vi "Scripting_SaveUpdateSubVIs.vi"(8 "error in (no error)":errorcluster, 11 "VI Refnum":refnum<vi>) -> (0 "error out":errorcluster)   [LabVIEW 2014]
uses:
  <vilib>/Utility/traverseref.llb/TRef TravTarget.ctl
  <vilib>/Utility/traverseref.llb/VI Scripting - Traverse.lvlib
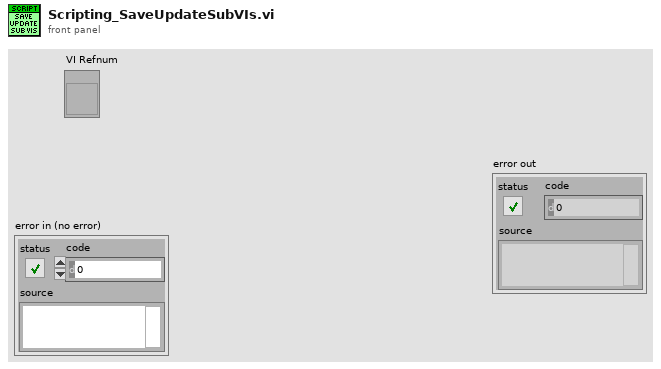
[diagram p1: front panel]
types:
  T1 = typedef "TRef TravTarget.ctl" = enum16{"FP", "BD", "Other"}
  T2 = enum32{"invalid lock state", "Not Locked", "Locked (No Password)", "Password-protected"}
  T3 = enum32{"not a typedef", "typedef", "strict typedef", "class private data"}
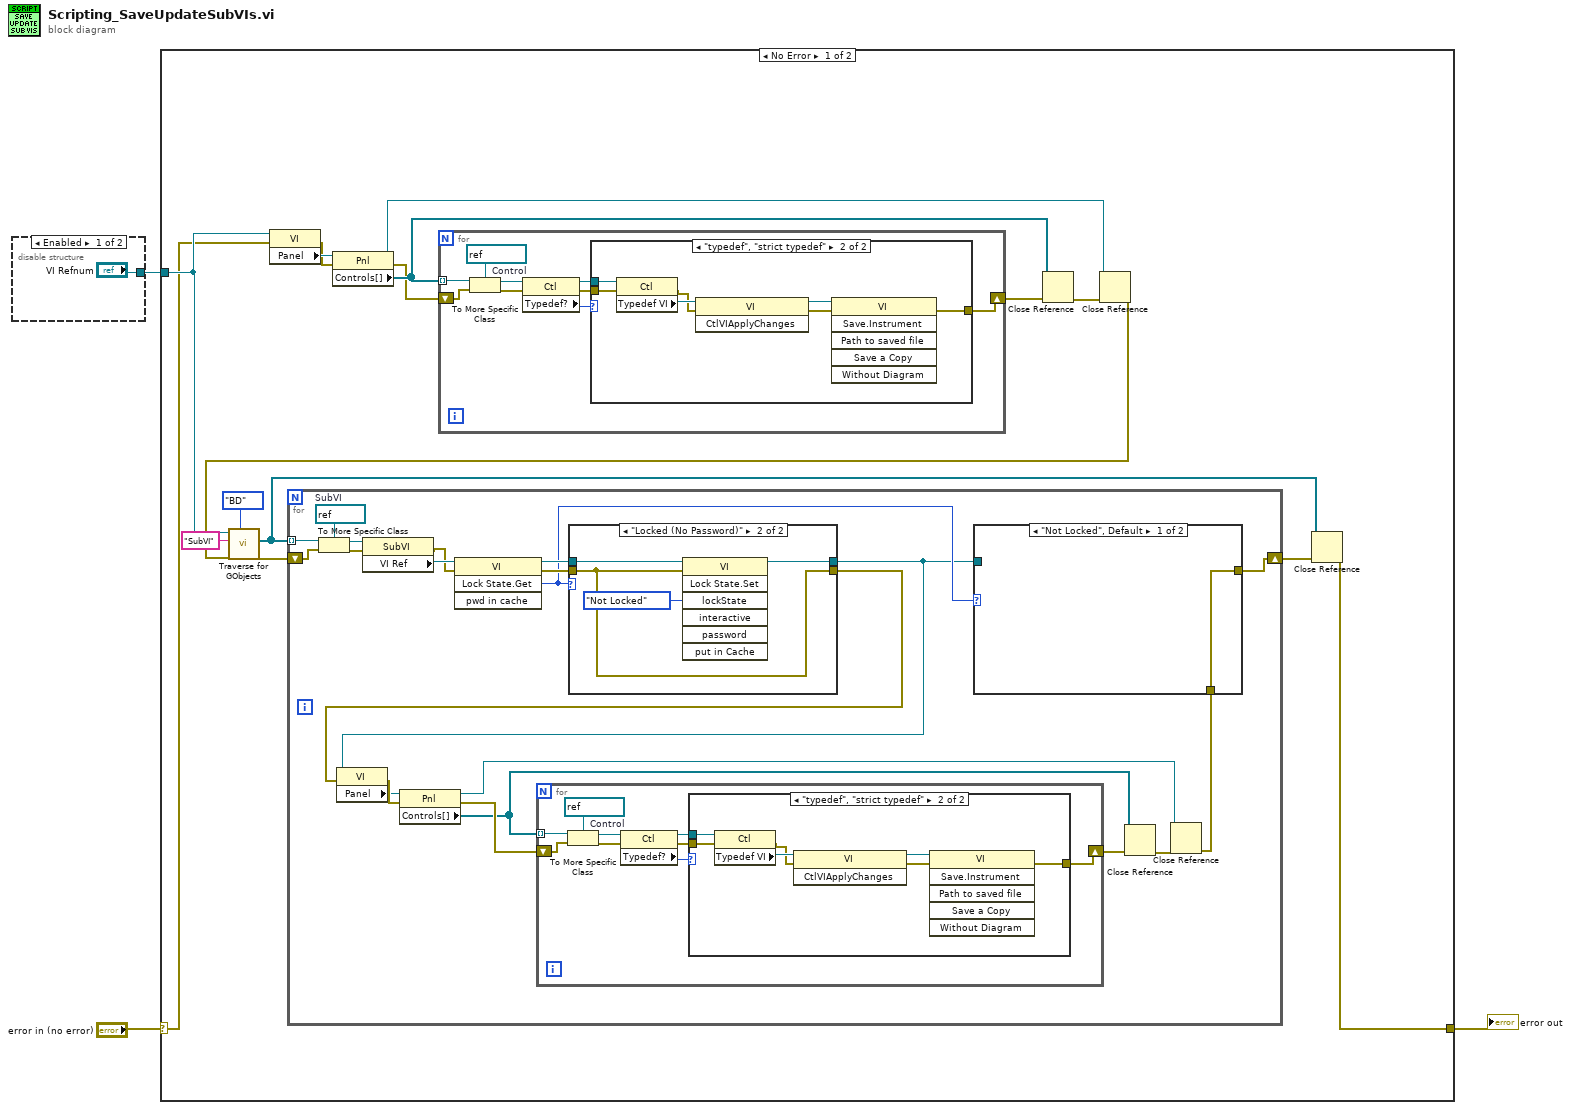
[diagram p0: block diagram]
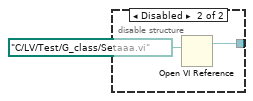
[diagram p2: hidden frame]
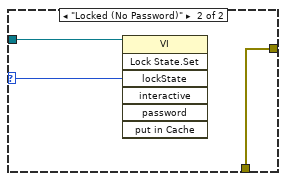
[diagram p3: hidden frame]
diagram:
  n1 = disable-structure shown="Enabled" {
    disable-tunnel: ["VI Refnum" w6] -> w1
    frame Enabled {
    }
    frame Disabled {
      n2 = Open VI Reference(vi path=path "C:/LV/Test/G_class/Setaaa.vi") -> (vi reference=w6:refnum<vi>)  [unwired: 5 in, 1 out]
    }
  }
  n3 = case shown="No Error" "error in (no error)" {
    selector: "error in (no error)" -> [w10 w88]
    tunnel: [w16 w88] -> w2
    tunnel: w1 -> [w15 _]
    frame No Error {
      n4 = property class="VI"(reference=w15, error in=w10) -> (error out=w11:errorcluster, "Panel"=w14:refnum<vi>)  [unwired: 1 out]
      n5 = property class="Pnl"(reference=w14, error in=w11) -> (reference out=w9:refnum<vi>, error out=w12:errorcluster, "Controls[]"=w13:refnum<vi>[])
      n6 = for {
        tunnel: w13 -> [w78] mode=indexing
        shift-right: [w71] -> w22
        shift-left: w12 -> [w75]
        w79 = refnum<vi> refnum  # Control
        n7 = To More Specific Class(target class=w79, reference=w78, error in=w75) -> (specific class reference=w77:refnum<vi>, error out=w76:errorcluster)
        n8 = property class="Ctl"(reference=w77, error in=w76) -> (reference out=w73:refnum<vi>, error out=w72:errorcluster, "Typedef?"=w74:T3)
        n9 = case shown="\"typedef\", \"strict typedef\"" w74 {
          tunnel: w73 -> [_ w87]
          tunnel: w72 -> [w80 w86]
          tunnel: [w80 w81] -> w71
          frame "not a typedef", Default {
          }
          frame "typedef", "strict typedef" {
            n10 = property class="Ctl"(reference=w87, error in=w86) -> (error out=w82:errorcluster, "Typedef VI"=w85:refnum<vi>)  [unwired: 1 out]
            n11 = invoke class="VI" method="CtlVIApplyChanges"(reference=w85, error in=w82) -> (reference out=w84:refnum<vi>, error out=w83:errorcluster)  [unwired: 1 in, 1 out]
            n12 = invoke class="VI" method="Save.Instrument"(reference=w84, error in=w83) -> (error out=w81:errorcluster)  [unwired: 4 in, 5 out]
          }
        }
      }
      n13 = Close Reference(reference=w13, error in (no error)=w22) -> (error out=w8:errorcluster)
      n14 = Close Reference(reference=w9, error in (no error)=w8) -> (error out=w7:errorcluster)
      n15 = call <vilib>:"Traverse for GObjects.vi"("Traverse Target"=TRef_TravTarget."BD", "error in (no error)"=w7, "Class Name"="SubVI", "VI Refnum"=w15) -> ("error out"=w19:errorcluster, "References"=w21:refnum<vi>[])  [unwired: 4 in, 2 out]
      n16 = for {
        tunnel: w21 -> [w42] mode=indexing
        shift-right: [w32] -> w20
        shift-left: w19 -> [w41]
        w43 = refnum<vi> refnum  # SubVI
        n17 = To More Specific Class(target class=w43, reference=w42, error in=w41) -> (specific class reference=w40:refnum<vi>, error out=w39:errorcluster)
        n18 = property class="SubVI"(reference=w40, error in=w39) -> (error out=w36:errorcluster, "VI Ref"=w38:refnum<vi>)  [unwired: 1 out]
        n19 = invoke class="VI" method="Lock State.Get"(reference=w38, error in=w36) -> (reference out=w37:refnum<vi>, error out=w35:errorcluster, "Get Lock State"=w33:T2)  [unwired: 2 in, 1 out]
        n20 = case shown="\"Locked (No Password)\"" w33 {
          tunnel: w37 -> [w65 w70]
          tunnel: w35 -> [w66 w67]
          tunnel: [w65 w68] -> w26
          tunnel: [w66 w67] -> w29
          frame "Not Locked", Default {
          }
          frame "Locked (No Password)" {
            n21 = invoke class="VI" method="Lock State.Set"(reference=w70, error in=w67, "lockState"=T2."Not Locked" ("Lock State")) -> (reference out=w68:refnum<vi>)  [unwired: 4 in, 6 out]
          }
        }
        n22 = property class="VI"(reference=w26, error in=w29) -> (error out=w31:errorcluster, "Panel"=w30:refnum<vi>)  [unwired: 1 out]
        n23 = property class="Pnl"(reference=w30, error in=w31) -> (reference out=w23:refnum<vi>, error out=w28:errorcluster, "Controls[]"=w27:refnum<vi>[])
        n24 = for {
          tunnel: w27 -> [w55] mode=indexing
          shift-right: [w48] -> w34
          shift-left: w28 -> [w52]
          w56 = refnum<vi> refnum  # Control
          n25 = To More Specific Class(target class=w56, reference=w55, error in=w52) -> (specific class reference=w54:refnum<vi>, error out=w53:errorcluster)
          n26 = property class="Ctl"(reference=w54, error in=w53) -> (reference out=w50:refnum<vi>, error out=w49:errorcluster, "Typedef?"=w51:T3)
          n27 = case shown="\"typedef\", \"strict typedef\"" w51 {
            tunnel: w50 -> [_ w64]
            tunnel: w49 -> [w57 w63]
            tunnel: [w57 w58] -> w48
            frame "not a typedef", Default {
            }
            frame "typedef", "strict typedef" {
              n28 = property class="Ctl"(reference=w64, error in=w63) -> (error out=w59:errorcluster, "Typedef VI"=w62:refnum<vi>)  [unwired: 1 out]
              n29 = invoke class="VI" method="CtlVIApplyChanges"(reference=w62, error in=w59) -> (reference out=w61:refnum<vi>, error out=w60:errorcluster)  [unwired: 1 in, 1 out]
              n30 = invoke class="VI" method="Save.Instrument"(reference=w61, error in=w60) -> (error out=w58:errorcluster)  [unwired: 4 in, 5 out]
            }
          }
        }
        n31 = Close Reference(reference=w27, error in (no error)=w34) -> (error out=w25:errorcluster)
        n32 = Close Reference(reference=w23, error in (no error)=w25) -> (error out=w24:errorcluster)
        n33 = case shown="\"Not Locked\", Default" w33 {
          selector: w33 -> [_ w46]
          tunnel: w26 -> [_ w47]
          tunnel: [w44 w45] -> w32
          tunnel: w24 -> [w44 w45]
          frame "Not Locked", Default {
          }
          frame "Locked (No Password)" {
            n34 = invoke class="VI" method="Lock State.Set"(reference=w47, "lockState"=w46) -> ()  [unwired: 5 in, 7 out]
          }
        }
      }
      n35 = Close Reference(reference=w21, error in (no error)=w20) -> (error out=w16:errorcluster)
    }
    frame Error {
    }
  }
  "error out" <- w2
